vi "软件版本号读取.vi"(8 "error in":errorcluster caption="错误输入", 11 "Channel":u16=81 format="%.0x") -> (0 "error out":errorcluster caption="错误输出", 3 "软件版本号":u32)   [LabVIEW 2020]
uses:
  <userlib>/PCANBasic/PCANBasic.lvlib
panel:
  out "function return 2":u32 format="%.0x"
  out "function return 3":u32 format="%.0x"
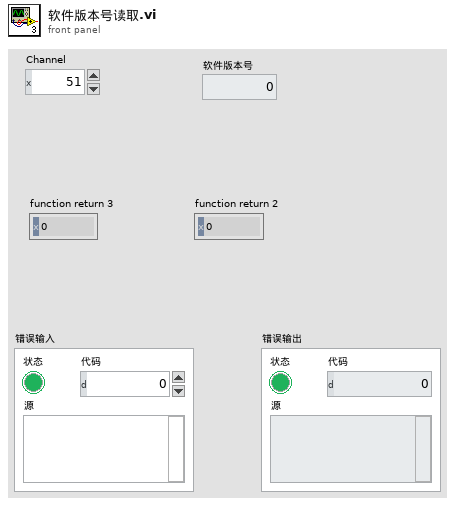
[diagram p1: front panel]
types:
  T1 = typedef "PCANBasic.lvlib/TPCANStatus.ctl" = u32
  T2 = typedef "PCANBasic.lvlib/TPCANMsgFD.ctl" = cluster{"ID":u32, "MSGTYPE":u8, "DLC":u8, "DATA":cluster{"[0]":u8, "[1]":u8, "[2]":u8, "[3]":u8, "[4]":u8, "[5]":u8, "[6]":u8, "[7]":u8, "[8]":u8, "[9]":u8, "[10]":u8, "[11]":u8, "[12]":u8, "[13]":u8, "[14]":u8, "[15]":u8, "[16]":u8, "[17]":u8, "[18]":u8, "[19]":u8, "[20]":u8, "[21]":u8, "[22]":u8, "[23]":u8, "[24]":u8, "[25]":u8, "[26]":u8, "[27]":u8, "[28]":u8, "[29]":u8, "[30]":u8, "[31]":u8, "[32]":u8, "[33]":u8, "[34]":u8, "[35]":u8, "[36]":u8, "[37]":u8, "[38]":u8, "[39]":u8, "[40]":u8, "[41]":u8, "[42]":u8, "[43]":u8, "[44]":u8, "[45]":u8, "[46]":u8, "[47]":u8, "[48]":u8, "[49]":u8, "[50]":u8, "[51]":u8, "[52]":u8, "[53]":u8, "[54]":u8, "[55]":u8, "[56]":u8, "[57]":u8, "[58]":u8, "[59]":u8, "[60]":u8, "[61]":u8, "[62]":u8, "[63]":u8}}
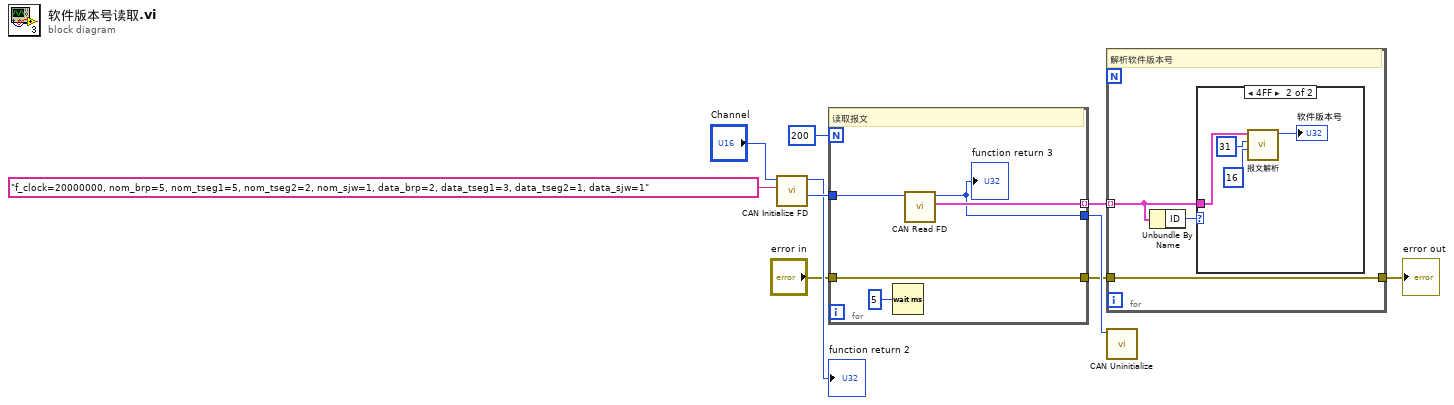
[diagram p0: block diagram]
diagram:
  n1 = call <userlib>:"CAN Initialize FD.vi"("BitrateFD"="f_clock=20000000, nom_brp=5, nom_tseg1=5, nom_tseg2=2, nom_sjw=1, data_brp=2, data_tseg1=3, data_tseg2=1, data_sjw=1", "Channel"="Channel") -> ("Channel out"=w7:u16, "TCANStatus"=→"function return 2":T1)  [unwired: 6 in, 2 out]
  n2 = for {
    N: 200 -> [_]
    tunnel: [w14] -> w4 mode=indexing
    tunnel: w7 -> [w13]
    tunnel: [w12] -> w5
    tunnel: "error in" -> [w11]
    tunnel: [w11] -> w2
    # "读取报文"
    n3 = Wait (ms)(milliseconds to wait=u32 5 ("等待时间（毫秒）")) -> ()  [unwired: 1 out]
    n4 = call <userlib>:"CAN Read FD.vi"("Channel"=w13) -> ("MessageBuffer out"=w14:T2, "TCANStatus"=w12:T1)  [unwired: 7 in, 2 out]
    "function return 3" <- w12
  }
  n5 = for {
    tunnel: w4 -> [w17] mode=indexing
    tunnel: w2 -> [w16]
    tunnel: [w16] -> w1
    # "解析软件版本号"
    n6 = Unbundle By Name(w17) -> ("ID"=w18:u32)
    n7 = case shown="4FF" w18 {
      tunnel: w17 -> [_ w19]
      frame 0, Default {
      }
      frame 1279 {
        n8 = call "报文解析.vi"("长度"=16, "起始位"=31, "MessageBuffer in"=w19) -> ("数字"=→"软件版本号":u32)  [unwired: 8 in]
      }
    }
  }
  "error out" <- w1
  n9 = call <userlib>:"CAN Uninitialize.vi"("Channel"=w5) -> ()  [unwired: 9 in, 2 out]
